vi "LEBITplc.SetPLCLL.vi"(0 "i ref in":refnum<vi>, 1 "Binary Selection":i16, 2 "i attribute in":T1, 3 "Value":dbl, 4 "index of element":i32, 5 "error IO":errorcluster) -> (14 "i ref out":refnum<vi>, 15 "i attribute out":T1, 19 "error out":errorcluster)   [LabVIEW 2014, in "LEBITplc.lvlib"]
uses:
  LEBITplc.lvlib
  LEBITplc.i attribute.ctl
  CSlibraries/UtilityLib/UtilityLib.valueStatus.ctl
  CSlibraries-extern/DimLVEvent/LVDimInterface/LVDimInterface.lvlib
  CSCore/CSSystem/CoreLib/CoreLib.lvlib
  CSlibraries/UtilityLib/UtilityLib.lvlib
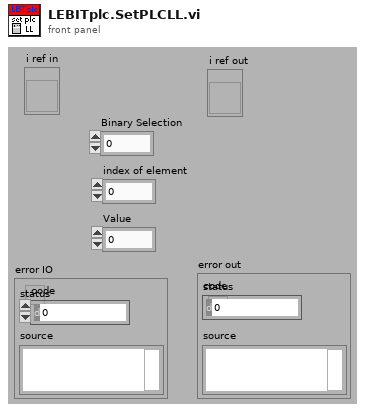
[diagram p1: front panel]
types:
  T1 = typedef "LEBITplc.lvlib/LEBITplc.i attribute.ctl" = cluster{"LLFLocation":string, "SetFileLocation":string, "nickNames":string[], "setValuePLCServiceID":i32[], "GUIServiceID":i32[], "monValuePLC":string[], "SetValueServiceID":i32[], "MonValueServiceID":i32[], "SetValue":dbl[][], "SetValueMin":dbl[], "SetValueMax":dbl[], "SetValueInfoServiceID":i32[], "GUINames":string[], "ListOfBases":string[], "Scale":dbl[], "Offset":dbl[], "setValuePLC":string[], "BaseName":string[], "ScaleServiceID":i32[], "OffsetServiceID":i32[], "AllPLCValues":string[], "CondSpecialArray":string[][], "CondSpecialIndex":i32[], "CondSpecialMonValue":dbl[], "RecentlyChanged":i32[], "SetFileLocationID":i32, "Dependent-Monitors":string[][], "LastLoadedFiles":string[], "IonGuideCalibLocation":string, "Monitor Dependent":string[], "Special":string[], "PLC?":bool[], "Start Date":string, "ListOfBasesServiceID":i32, "SETRA VISA resource":refnum<visa-resource-name>}
  T2 = typedef "UtilityLib.lvlib/UtilityLib.valueStatus.ctl" = enum16{"no info available", "stand by/off", "on", "warning", "alarm/malfunction", "not implemented", "user action required", "important information", "system default", "control default", "indicator default", "button default"}
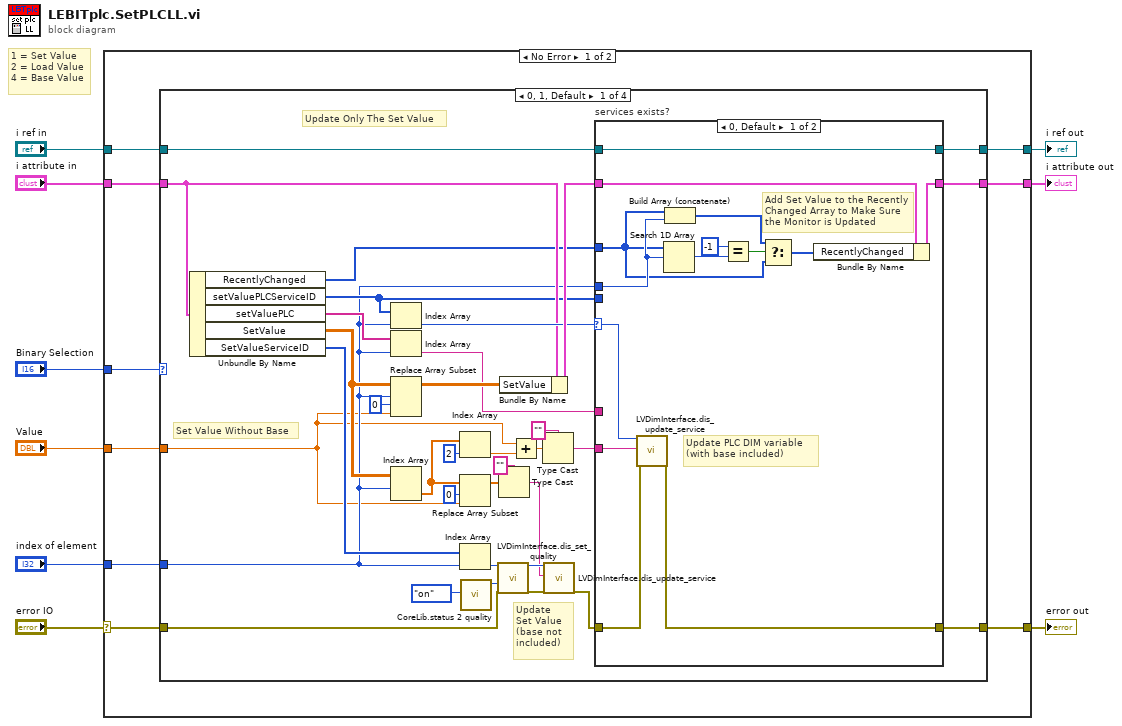
[diagram p0: block diagram]
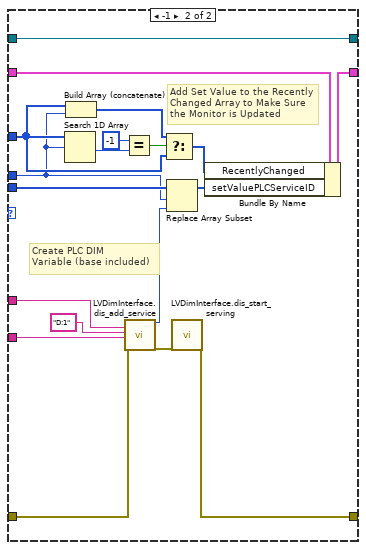
[diagram p2: hidden frame]
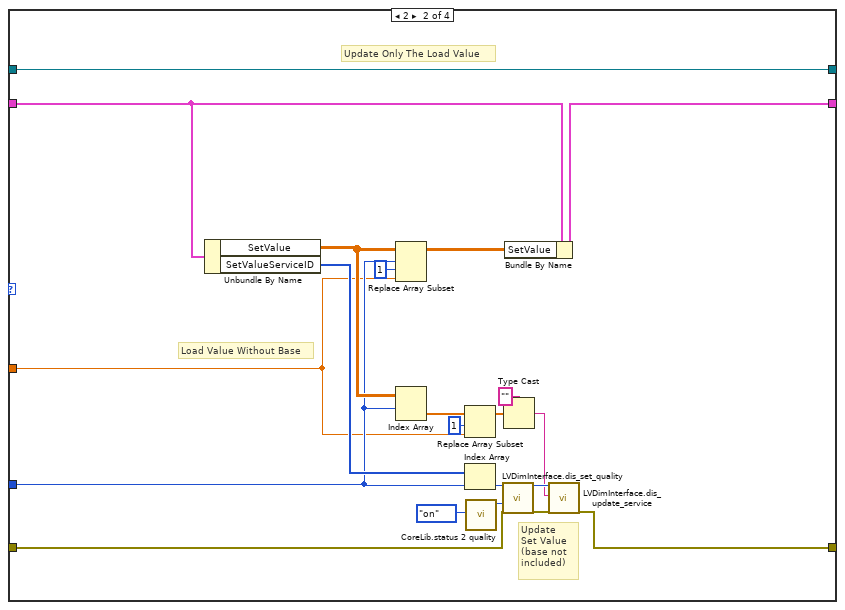
[diagram p3: hidden frame]
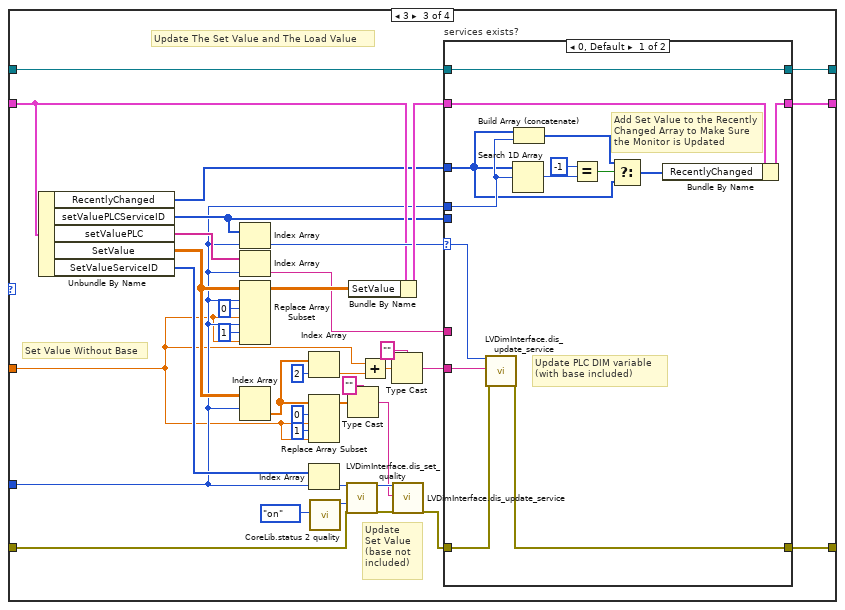
[diagram p4: hidden frame]
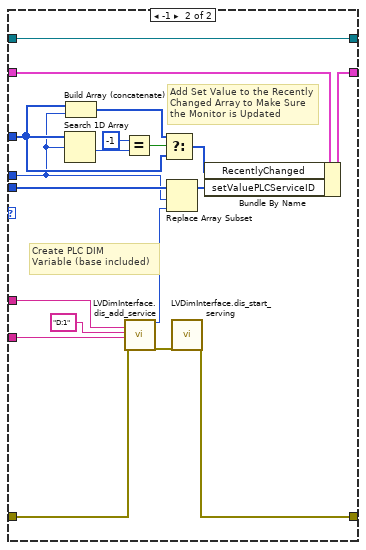
[diagram p5: hidden frame]
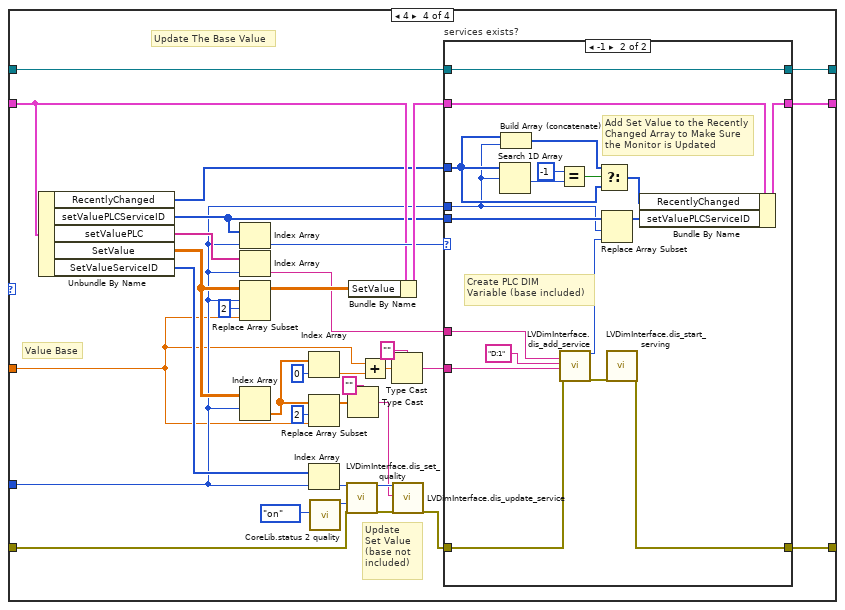
[diagram p6: hidden frame]
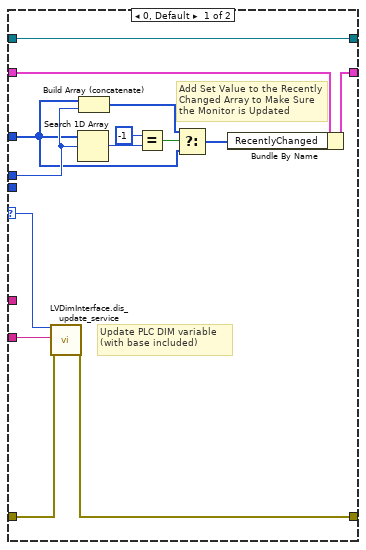
[diagram p7: hidden frame]
diagram:
  # "1 = Set Value\n2 = Load Value\n4 = Base Value"
  n1 = case shown="No Error" "error IO" {
    selector: "error IO" -> [w14 w243]
    tunnel: "index of element" -> [w11 _]
    tunnel: "i attribute in" -> [w13 w244]
    tunnel: [w18 w244] -> w7
    tunnel: [w17 w243] -> w6
    tunnel: [w16 w245] -> w5
    tunnel: "i ref in" -> [w15 w245]
    tunnel: "Value" -> [w12 _]
    tunnel: "Binary Selection" -> [w10 _]
    frame No Error {
      n2 = case shown="0, 1, Default" w10 {
        tunnel: [w45 w87 w135 w202] -> w18
        tunnel: [w44 w86 w134 w201] -> w17
        tunnel: [w43 w88 w133 w200] -> w16
        tunnel: w15 -> [w41 w88 w131 w198]
        tunnel: w14 -> [w36 w98 w126 w193]
        tunnel: w13 -> [w35 w97 w125 w192]
        tunnel: w12 -> [w19 w89 w107 w176]
        tunnel: w11 -> [w24 w91 w110 w177]
        frame 0, 1, Default {
          # "Set Value Without Base"
          # "Update Only The Set Value"
          # "Update\nSet Value \n(base not included)"
          n3 = Unbundle By Name(w35) -> ("RecentlyChanged"=w25:i32[], "setValuePLCServiceID"=w34:i32[], "setValuePLC"=w33:string[], "SetValue"=w30:dbl[][], "SetValueServiceID"=w32:i32[])
          n4 = Index Array(array=w34, index=w24) -> (element=w39:i32)
          n5 = Index Array(array=w33, index=w24) -> (element=w40:string)
          n6 = Replace Array Subset(array=w30, new element=w19, index (row)=w24, index (col)=0 ("disabled index (col)")) -> (w52:dbl[][])
          n7 = Index Array(array=w30, index (row)=w24) -> (element=w23:dbl[])  [unwired: 1 in]
          n8 = Index Array(array=w23, index=2) -> (element=w20:dbl)
          n9 = Replace Array Subset(array=w23, new element=w19, index=0) -> (w29:dbl[])
          n10 = Index Array(array=w32, index=w24) -> (element=w48:i32)
          n11 = call "CoreLib.status 2 quality.vi"("valueStatus"=UtilityLib.valueStatus."on") -> ("quality"=w49:i32)  [unwired: 18 in]
          n12 = call "LVDimInterface.dis_set_quality.vi"("my_serviceID"=w48, "quality"=w49, "error in (no error)"=w36) -> ("my_serviceID (out)"=w47:i32, "error out"=w46:errorcluster)  [unwired: 15 in]
          n13 = Type Cast(type="", x=w29) -> (*(type *) &x=w38:string)
          n14 = Bundle By Name(cluster=w35, "SetValue"=w52) -> (w51:T1)
          n15 = Add(x=w19, y=w20) -> (x+y=w21:dbl)
          n16 = Type Cast(type="", x=w21) -> (*(type *) &x=w26:string)
          n17 = call "LVDimInterface.dis_update_service.vi"("my_serviceID"=w47, "data"=w38, "error in (no error)"=w46) -> ("error out"=w42:errorcluster)  [unwired: 14 in, 2 out]
          n18 = case "services exists?" shown="0, Default" w39 {
            selector: w39 -> [w57 _]
            tunnel: w26 -> [w66 w74]
            tunnel: w40 -> [_ w75]
            tunnel: w41 -> [w65 w81]
            tunnel: [w65 w81] -> w43
            tunnel: w42 -> [w64 w79]
            tunnel: w34 -> [_ w85]
            tunnel: [w63 w77] -> w44
            tunnel: w24 -> [w56 w67]
            tunnel: w51 -> [w54 w82]
            tunnel: [w53 w80] -> w45
            tunnel: w25 -> [w55 w69]
            frame 0, Default {
              # "Add Set Value to the Recently \nChanged Array to Make Sure the Monitor is Updated"
              # "Update PLC DIM variable\n(with base included)"
              n19 = call "LVDimInterface.dis_update_service.vi"("my_serviceID"=w57, "data"=w66, "error in (no error)"=w64) -> ("error out"=w63:errorcluster)  [unwired: 14 in, 2 out]
              n20 = Search 1D Array(1D array=w55, element=w56) -> (index of element=w62:i32)  [unwired: 1 in]
              n21 = Build Array (concatenate)(w55, w56) -> (w58:i32[])
              n22 = Equal?(x=-1, y=w62) -> (x = y?=w60:bool)
              n23 = Select(t=w58, s=w60, f=w55) -> (s? t:f=w59:i32[])
              n24 = Bundle By Name(cluster=w54, "RecentlyChanged"=w59) -> (w53:T1)
            }
            frame -1 {
              # "Add Set Value to the Recently \nChanged Array to Make Sure the Monitor is Updated"
              # "Create PLC DIM\nVariable (base included)"
              n25 = Search 1D Array(1D array=w69, element=w67) -> (index of element=w73:i32)  [unwired: 1 in]
              n26 = Build Array (concatenate)(w69, w67) -> (w68:i32[])
              n27 = Equal?(x=-1, y=w73) -> (x = y?=w71:bool)
              n28 = call "LVDimInterface.dis_add_service.vi"("serviceName"=w75, "typeDescriptor"="D:1", "data"=w74, "error in (no error)"=w79) -> ("my_serviceID"=w84:i32, "error out"=w78:errorcluster)  [unwired: 14 in]
              n29 = Select(t=w68, s=w71, f=w69) -> (s? t:f=w70:i32[])
              n30 = Replace Array Subset(array=w85, new element=w84, index=w67) -> (w83:i32[])
              n31 = call "LVDimInterface.dis_start_serving.vi"("error in (no error)"=w78) -> ("error out"=w77:errorcluster)  [unwired: 17 in, 1 out]
              n32 = Bundle By Name(cluster=w82, "RecentlyChanged"=w70, "setValuePLCServiceID"=w83) -> (w80:T1)
            }
          }
        }
        frame 2 {
          # "Load Value Without Base"
          # "Update Only The Load Value"
          # "Update\nSet Value \n(base not included)"
          n33 = Unbundle By Name(w97) -> ("SetValue"=w94:dbl[][], "SetValueServiceID"=w96:i32[])
          n34 = Replace Array Subset(array=w94, new element=w89, index (row)=w91, index (col)=1 ("disabled index (col)")) -> (w106:dbl[][])
          n35 = Index Array(array=w94, index (row)=w91) -> (element=w90:dbl[])  [unwired: 1 in]
          n36 = Replace Array Subset(array=w90, new element=w89, index=1) -> (w93:dbl[])
          n37 = Index Array(array=w96, index=w91) -> (element=w103:i32)
          n38 = call "CoreLib.status 2 quality.vi"("valueStatus"=UtilityLib.valueStatus."on") -> ("quality"=w104:i32)  [unwired: 18 in]
          n39 = call "LVDimInterface.dis_set_quality.vi"("my_serviceID"=w103, "quality"=w104, "error in (no error)"=w98) -> ("my_serviceID (out)"=w102:i32, "error out"=w101:errorcluster)  [unwired: 15 in]
          n40 = Type Cast(type="", x=w93) -> (*(type *) &x=w100:string)
          n41 = Bundle By Name(cluster=w97, "SetValue"=w106) -> (w87:T1)
          n42 = call "LVDimInterface.dis_update_service.vi"("my_serviceID"=w102, "data"=w100, "error in (no error)"=w101) -> ("error out"=w86:errorcluster)  [unwired: 14 in, 2 out]
        }
        frame 3 {
          # "Set Value Without Base"
          # "Update The Set Value and The Load Value"
          # "Update\nSet Value \n(base not included)"
          n43 = Unbundle By Name(w125) -> ("RecentlyChanged"=w115:i32[], "setValuePLCServiceID"=w124:i32[], "setValuePLC"=w123:string[], "SetValue"=w120:dbl[][], "SetValueServiceID"=w122:i32[])
          n44 = Index Array(array=w124, index=w110) -> (element=w129:i32)
          n45 = Index Array(array=w123, index=w110) -> (element=w130:string)
          n46 = Replace Array Subset(array=w120, new element #1=w107, index (row) #1=w110, index (col) #1=0 ("disabled index (col)"), new element #2=w107, index (row) #2=w110, index (col) #2=1 ("disabled index (col)")) -> (w142:dbl[][])
          n47 = Index Array(array=w120, index (row)=w110) -> (element=w114:dbl[])  [unwired: 1 in]
          n48 = Index Array(array=w114, index=2) -> (element=w111:dbl)
          n49 = Replace Array Subset(array=w114, new element #1=w107, index #1=0 ("index"), new element #2=w107, index #2=1 ("index")) -> (w119:dbl[])
          n50 = Index Array(array=w122, index=w110) -> (element=w138:i32)
          n51 = call "CoreLib.status 2 quality.vi"("valueStatus"=UtilityLib.valueStatus."on") -> ("quality"=w139:i32)  [unwired: 18 in]
          n52 = call "LVDimInterface.dis_set_quality.vi"("my_serviceID"=w138, "quality"=w139, "error in (no error)"=w126) -> ("my_serviceID (out)"=w137:i32, "error out"=w136:errorcluster)  [unwired: 15 in]
          n53 = Type Cast(type="", x=w119) -> (*(type *) &x=w128:string)
          n54 = Bundle By Name(cluster=w125, "SetValue"=w142) -> (w141:T1)
          n55 = Add(x=w107, y=w111) -> (x+y=w112:dbl)
          n56 = Type Cast(type="", x=w112) -> (*(type *) &x=w116:string)
          n57 = call "LVDimInterface.dis_update_service.vi"("my_serviceID"=w137, "data"=w128, "error in (no error)"=w136) -> ("error out"=w132:errorcluster)  [unwired: 14 in, 2 out]
          n58 = case "services exists?" shown="0, Default" w129 {
            selector: w129 -> [w147 _]
            tunnel: w116 -> [w156 w164]
            tunnel: w130 -> [_ w165]
            tunnel: w131 -> [w155 w171]
            tunnel: [w155 w171] -> w133
            tunnel: w132 -> [w154 w169]
            tunnel: w124 -> [_ w175]
            tunnel: [w153 w167] -> w134
            tunnel: w110 -> [w146 w157]
            tunnel: w141 -> [w144 w172]
            tunnel: [w143 w170] -> w135
            tunnel: w115 -> [w145 w159]
            frame 0, Default {
              # "Add Set Value to the Recently \nChanged Array to Make Sure the Monitor is Updated"
              # "Update PLC DIM variable\n(with base included)"
              n59 = call "LVDimInterface.dis_update_service.vi"("my_serviceID"=w147, "data"=w156, "error in (no error)"=w154) -> ("error out"=w153:errorcluster)  [unwired: 14 in, 2 out]
              n60 = Search 1D Array(1D array=w145, element=w146) -> (index of element=w152:i32)  [unwired: 1 in]
              n61 = Build Array (concatenate)(w145, w146) -> (w148:i32[])
              n62 = Equal?(x=-1, y=w152) -> (x = y?=w150:bool)
              n63 = Select(t=w148, s=w150, f=w145) -> (s? t:f=w149:i32[])
              n64 = Bundle By Name(cluster=w144, "RecentlyChanged"=w149) -> (w143:T1)
            }
            frame -1 {
              # "Add Set Value to the Recently \nChanged Array to Make Sure the Monitor is Updated"
              # "Create PLC DIM\nVariable (base included)"
              n65 = Search 1D Array(1D array=w159, element=w157) -> (index of element=w163:i32)  [unwired: 1 in]
              n66 = Build Array (concatenate)(w159, w157) -> (w158:i32[])
              n67 = Equal?(x=-1, y=w163) -> (x = y?=w161:bool)
              n68 = call "LVDimInterface.dis_add_service.vi"("serviceName"=w165, "typeDescriptor"="D:1", "data"=w164, "error in (no error)"=w169) -> ("my_serviceID"=w174:i32, "error out"=w168:errorcluster)  [unwired: 14 in]
              n69 = Select(t=w158, s=w161, f=w159) -> (s? t:f=w160:i32[])
              n70 = Replace Array Subset(array=w175, new element=w174, index=w157) -> (w173:i32[])
              n71 = call "LVDimInterface.dis_start_serving.vi"("error in (no error)"=w168) -> ("error out"=w167:errorcluster)  [unwired: 17 in, 1 out]
              n72 = Bundle By Name(cluster=w172, "RecentlyChanged"=w160, "setValuePLCServiceID"=w173) -> (w170:T1)
            }
          }
        }
        frame 4 {
          # "Value Base"
          # "Update The Base Value"
          # "Update\nSet Value \n(base not included)"
          n73 = Unbundle By Name(w192) -> ("RecentlyChanged"=w182:i32[], "setValuePLCServiceID"=w191:i32[], "setValuePLC"=w190:string[], "SetValue"=w187:dbl[][], "SetValueServiceID"=w189:i32[])
          n74 = Index Array(array=w191, index=w177) -> (element=w196:i32)
          n75 = Index Array(array=w190, index=w177) -> (element=w197:string)
          n76 = Replace Array Subset(array=w187, new element=w176, index (row)=w177, index (col)=2 ("disabled index (col)")) -> (w209:dbl[][])
          n77 = Index Array(array=w187, index (row)=w177) -> (element=w181:dbl[])  [unwired: 1 in]
          n78 = Index Array(array=w181, index=0) -> (element=w178:dbl)
          n79 = Replace Array Subset(array=w181, new element=w176, index=2) -> (w186:dbl[])
          n80 = Index Array(array=w189, index=w177) -> (element=w205:i32)
          n81 = call "CoreLib.status 2 quality.vi"("valueStatus"=UtilityLib.valueStatus."on") -> ("quality"=w206:i32)  [unwired: 18 in]
          n82 = call "LVDimInterface.dis_set_quality.vi"("my_serviceID"=w205, "quality"=w206, "error in (no error)"=w193) -> ("my_serviceID (out)"=w204:i32, "error out"=w203:errorcluster)  [unwired: 15 in]
          n83 = Type Cast(type="", x=w186) -> (*(type *) &x=w195:string)
          n84 = Bundle By Name(cluster=w192, "SetValue"=w209) -> (w208:T1)
          n85 = Add(x=w176, y=w178) -> (x+y=w179:dbl)
          n86 = Type Cast(type="", x=w179) -> (*(type *) &x=w183:string)
          n87 = call "LVDimInterface.dis_update_service.vi"("my_serviceID"=w204, "data"=w195, "error in (no error)"=w203) -> ("error out"=w199:errorcluster)  [unwired: 14 in, 2 out]
          n88 = case "services exists?" shown="-1" w196 {
            selector: w196 -> [w214 _]
            tunnel: w183 -> [w223 w231]
            tunnel: w197 -> [_ w232]
            tunnel: w198 -> [w222 w238]
            tunnel: [w222 w238] -> w200
            tunnel: w199 -> [w221 w236]
            tunnel: w191 -> [_ w242]
            tunnel: [w220 w234] -> w201
            tunnel: w177 -> [w213 w224]
            tunnel: w208 -> [w211 w239]
            tunnel: [w210 w237] -> w202
            tunnel: w182 -> [w212 w226]
            frame 0, Default {
              # "Add Set Value to the Recently \nChanged Array to Make Sure the Monitor is Updated"
              # "Update PLC DIM variable\n(with base included)"
              n89 = call "LVDimInterface.dis_update_service.vi"("my_serviceID"=w214, "data"=w223, "error in (no error)"=w221) -> ("error out"=w220:errorcluster)  [unwired: 14 in, 2 out]
              n90 = Search 1D Array(1D array=w212, element=w213) -> (index of element=w219:i32)  [unwired: 1 in]
              n91 = Build Array (concatenate)(w212, w213) -> (w215:i32[])
              n92 = Equal?(x=-1, y=w219) -> (x = y?=w217:bool)
              n93 = Select(t=w215, s=w217, f=w212) -> (s? t:f=w216:i32[])
              n94 = Bundle By Name(cluster=w211, "RecentlyChanged"=w216) -> (w210:T1)
            }
            frame -1 {
              # "Add Set Value to the Recently \nChanged Array to Make Sure the Monitor is Updated"
              # "Create PLC DIM\nVariable (base included)"
              n95 = Search 1D Array(1D array=w226, element=w224) -> (index of element=w230:i32)  [unwired: 1 in]
              n96 = Build Array (concatenate)(w226, w224) -> (w225:i32[])
              n97 = Equal?(x=-1, y=w230) -> (x = y?=w228:bool)
              n98 = call "LVDimInterface.dis_add_service.vi"("serviceName"=w232, "typeDescriptor"="D:1", "data"=w231, "error in (no error)"=w236) -> ("my_serviceID"=w241:i32, "error out"=w235:errorcluster)  [unwired: 14 in]
              n99 = Select(t=w225, s=w228, f=w226) -> (s? t:f=w227:i32[])
              n100 = Replace Array Subset(array=w242, new element=w241, index=w224) -> (w240:i32[])
              n101 = call "LVDimInterface.dis_start_serving.vi"("error in (no error)"=w235) -> ("error out"=w234:errorcluster)  [unwired: 17 in, 1 out]
              n102 = Bundle By Name(cluster=w239, "RecentlyChanged"=w227, "setValuePLCServiceID"=w240) -> (w237:T1)
            }
          }
        }
      }
    }
    frame Error {
    }
  }
  "i attribute out" <- w7
  "error out" <- w6
  "i ref out" <- w5
